vi "Handle.vi"(8 "error in (no error)":errorcluster, 11 "AG in":refnum<class "AG.lvclass">) -> (0 "error out":errorcluster, 3 "AG out":refnum<class "AG.lvclass">)   [LabVIEW 2018, in "AG.lvclass"]
uses:
  AG.lvclass
  AG.lvclass/AG.ctl
  Device/Device.lvclass/Device.ctl
  Device/angles/angles.lvclass
  C:/Users/observer/Desktop/Sparc4GUI/Versao ZeroMQ/SPARC4_GUI -20240706_20240708/Device/Device.lvclass
  Client/Client.lvclass
  Comm/Stream/Stream.lvclass
  Device/Device.lvclass
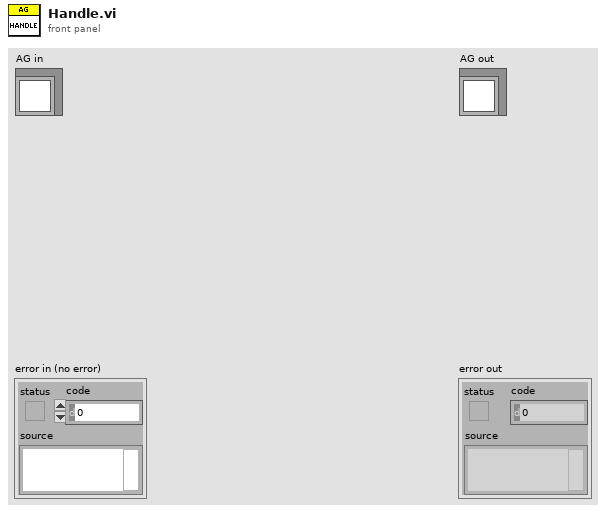
[diagram p1: front panel]
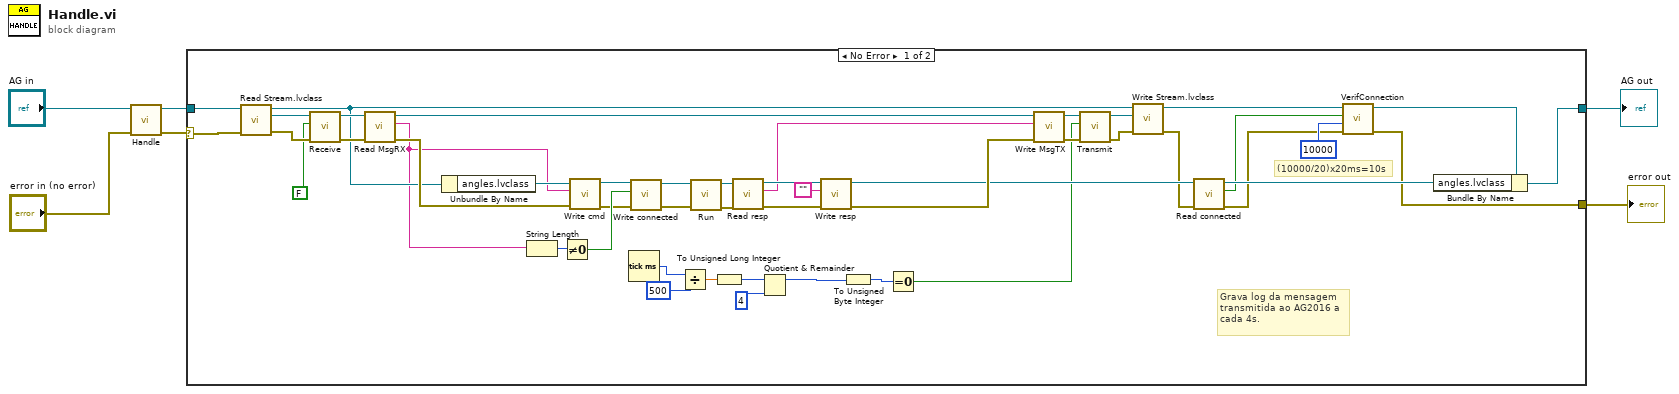
[diagram p0: block diagram]
diagram:
  n1 = call-parent "Handle.vi"("error in (no error)"="error in (no error)", "Client in"="AG in") -> ("error out"=w3:errorcluster, "Client out"=w4:refnum<class "AG.lvclass">)  [unwired: 8 in]
  n2 = case shown="No Error" w3 {
    selector: w3 -> [w51 w55]
    tunnel: [w22 w55] -> w1
    tunnel: [w50 w54] -> w2
    tunnel: w4 -> [w41 w54]
    frame No Error {
      # "Grava log da mensagem\ntransmitida ao AG2016 a\ncada 4s."
      # "(10000/20)x20ms=10s"
      n3 = call-dynamic "Read Stream.lvclass.vi"("error in (no error)"=w51, "Client in"=w41) -> ("error out"=w52:errorcluster, "Stream.lvclass"=w53:refnum<class "Stream.lvclass">, "Client out"=w43:refnum<class "AG.lvclass">)  [unwired: 7 in]
      n4 = call-dynamic "Receive.vi"("error in (no error)"=w52, "log?"=FALSE, "Stream in"=w53) -> ("error out"=w49:errorcluster, "Stream out"=w48:refnum<class "Stream.lvclass">)  [unwired: 7 in]
      n5 = call-dynamic "Read MsgRX.vi"("error in (no error)"=w49, "Comm in"=w48) -> ("error out"=w47:errorcluster, "MsgRX"=w33:string, "Comm out"=w27:refnum<class "Stream.lvclass">)  [unwired: 7 in]
      n6 = Unbundle By Name(w43) -> ("angles.lvclass"=w37:refnum<class "angles.lvclass">)
      n7 = String Length(string=w33) -> (length=w34:i32)
      n8 = Not Equal To 0?(x=w34) -> (x != 0?=w20:bool)
      n9 = call-dynamic "Write cmd.vi"("error in (no error)"=w47, "cmd"=w33, "Device in"=w37) -> ("error out"=w19:errorcluster, "Device out"=w18:refnum<class "angles.lvclass">)  [unwired: 7 in]
      n10 = Tick Count (ms)() -> (millisecond timer value=w14:u32)
      n11 = call "Write connected.vi"("error in (no error)"=w19, "connected"=w20, "Device in"=w18) -> ("error out"=w16:errorcluster, "Device out"=w17:refnum<class "angles.lvclass">)  [unwired: 7 in]
      n12 = Divide(x=w14, y=u32 500) -> (x/y=w9:dbl)
      n13 = call-dynamic "Run.vi"("error in (no error)"=w16, "angles in"=w17) -> ("error out"=w31:errorcluster, "angles out"=w32:refnum<class "angles.lvclass">)  [unwired: 8 in]
      n14 = To Unsigned Long Integer(number=w9) -> (unsigned 32bit integer=w8:u32)
      n15 = call-dynamic "Read resp.vi"("error in (no error)"=w31, "Device in"=w32) -> ("error out"=w39:errorcluster, "resp"=w36:string, "Device out"=w40:refnum<class "angles.lvclass">)  [unwired: 7 in]
      n16 = Quotient & Remainder(x=w8, y=u32 4) -> (x-y*floor(x/y)=w11:u32)  [unwired: 1 out]
      n17 = call-dynamic "Write resp.vi"("error in (no error)"=w39, "resp"="" ("cmd"), "Device in"=w40) -> ("error out"=w46:errorcluster, "Device out"=w30:refnum<class "angles.lvclass">)  [unwired: 7 in]
      n18 = To Unsigned Byte Integer(number=w11) -> (unsigned 8bit integer=w10:u8)
      n19 = Equal To 0?(x=w10) -> (x = 0?=w7:bool)
      n20 = call-dynamic "Write MsgTX.vi"("error in (no error)"=w46, "MsgTX"=w36, "Comm in"=w27) -> ("error out"=w44:errorcluster, "Comm out"=w45:refnum<class "Stream.lvclass">)  [unwired: 7 in]
      n21 = call-dynamic "Transmit.vi"("error in (no error)"=w44, "log?"=w7, "Stream in"=w45) -> ("error out"=w42:errorcluster, "Stream out"=w35:refnum<class "Stream.lvclass">)  [unwired: 7 in]
      n22 = call-dynamic "Write Stream.lvclass.vi"("error in (no error)"=w42, "Stream.lvclass"=w35, "Client in"=w43) -> ("error out"=w29:errorcluster, "Client out"=w26:refnum<class "AG.lvclass">)  [unwired: 7 in]
      n23 = call "Read connected.vi"("error in (no error)"=w29, "Device in"=w30) -> ("error out"=w23:errorcluster, "connected"=w25:bool, "Device out"=w28:refnum<class "angles.lvclass">)  [unwired: 7 in]
      n24 = call-dynamic "VerifConnection.vi"("error in (no error)"=w23, "timeout in ms (1000)"=u32 10000 ("period (ms)"), "device connected in"=w25, "Client in"=w26) -> ("error out"=w22:errorcluster, "Client out"=w21:refnum<class "AG.lvclass">)  [unwired: 6 in]
      n25 = Bundle By Name(cluster=w21, "angles.lvclass"=w28) -> (w50:refnum<class "AG.lvclass">)
    }
    frame Error {
    }
  }
  "error out" <- w1
  "AG out" <- w2
